vi "unRegisterTimer.vi"(8 "error in (no error)":errorcluster, 10 "Name":string, 11 "UserEventTimer in":refnum<class "TimerEngine.lvclass">) -> (0 "error out":errorcluster, 3 "UserEventTimer out":refnum<class "TimerEngine.lvclass">)   [LabVIEW 2017, in "TimerEngine.lvlib" / "TimerEngine.lvclass"]
uses:
  TimerEngine.lvclass
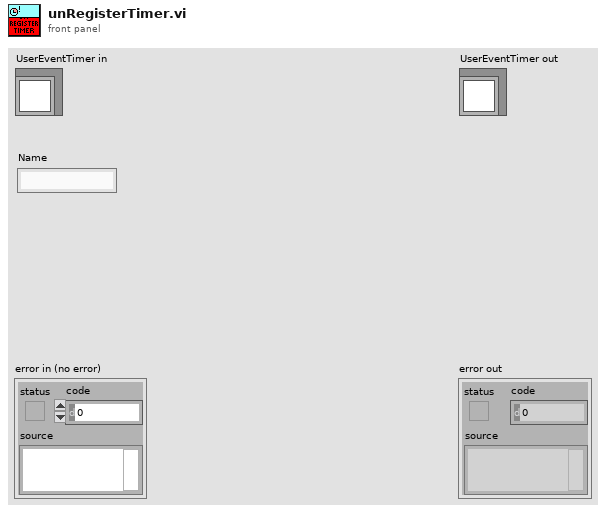
[diagram p1: front panel]
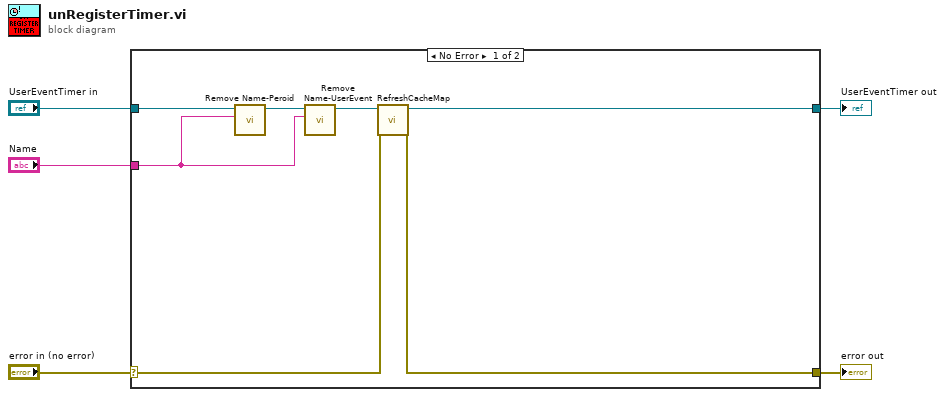
[diagram p0: block diagram]
diagram:
  n1 = case shown="No Error" "error in (no error)" {
    selector: "error in (no error)" -> [w7 w14]
    tunnel: [w6 w14] -> w4
    tunnel: [w8 w13] -> w2
    tunnel: "UserEventTimer in" -> [w12 w13]
    tunnel: "Name" -> [w10 _]
    frame No Error {
      n2 = call "Remove Name-Peroid.vi"("Name"=w10, "UserEventTimer in"=w12) -> ("UserEventTimer out"=w11:refnum<class "TimerEngine.lvclass">)  [unwired: 8 in, 1 out]
      n3 = call "Remove Name-UserEvent.vi"("Name"=w10, "UserEventTimer in"=w11) -> ("UserEventTimer out"=w9:refnum<class "TimerEngine.lvclass">)  [unwired: 9 in]
      n4 = call "RefreshCacheMap.vi"("error in (no error)"=w7, "UserEventTimer in"=w9) -> ("error out"=w6:errorcluster, "UserEventTimer out"=w8:refnum<class "TimerEngine.lvclass">)  [unwired: 8 in]
    }
    frame Error {
    }
  }
  "error out" <- w4
  "UserEventTimer out" <- w2
